vi "CPP-SolAEsaveTimeTraces.vi"() -> (5 "Plug in titles":string[](array[string]), 7 "Plug in values":string[](array[string]))   [LabVIEW 2021]
uses:
  Controls/File Header mode.ctl
  Globals/Meas_global.vi
panel:
  out "Data to save (ALL channels)":i32[](array[ring])
  # "Minimalist Save-All-Channels plugin, with options hard-coded to suit SolAE jobs\n\n\nYou Must have selected the \"Save Data\" option on the \nMeasurement Program for this vi to save time traces"
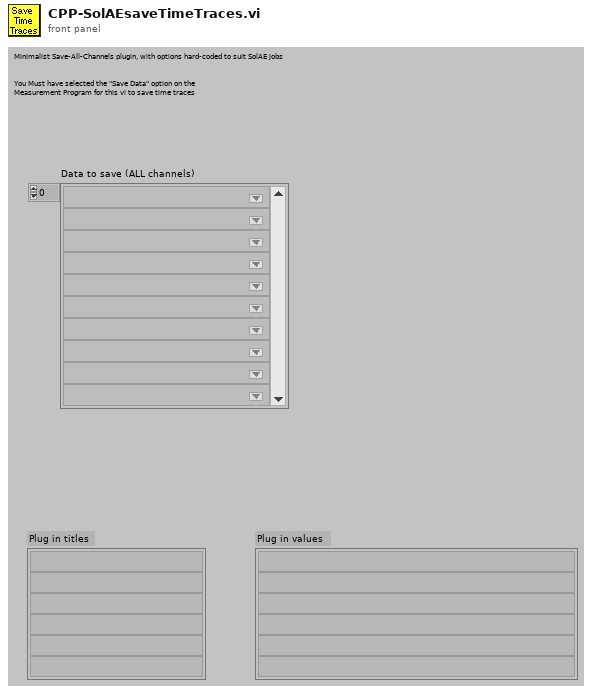
[diagram p1: front panel]
types:
  T1 = typedef "Analysis_info_cluster.ctl" = cluster{"Colour":u32, "Inst type":T2, "Inst name":string, "Symbol":string, "Code name":string, "Extra Info":string, "Inst Array":T3, "Extra Titles":string[], "Extra Values":string[], "U":dbl, "u^2":dbl, "u^3":dbl, "u^4":dbl, "Skew_u":dbl, "Kurt_u":dbl, "Sd Error in Mean":dbl, "% u'/U":dbl, "X":dbl, "Y":dbl, "Z":dbl, "Timescale integral Estimate":dbl, "Sd Error in Variance":dbl, "Calib File":path, "Calib Constants":dbl[], "Output Position":bool, "Stats":enum16{"None", "Basic", "Full"}, "Av Sampling Rate":dbl, "Av No of Samples":dbl, "Total Meas Time (s)":dbl, "ADAM Ch Name":string, "Max value":dbl, "Min value":dbl, "Req Sample Rate Hz":dbl, "Sync Delay Time (s)":dbl, "Ch No":i16, "Device":string, "Use Latest Calib":bool, "Port":string, "Metadata Ch Names":string[], "Metadata Ch Values":string[], "Label":string}
  T2 = typedef "Inst_type.ctl" = enum16{"Raw voltage", "Raw with zero offsetting", "Propeller anemometer", "Pressure Transducer", "Pitot-static tube", "Hot wire", "Cross wire 1", "Cross wire 2", "Generic Linear", "Generic Polynomial", "Generic BackPoly", "Fast FID", "Thermocouple", "Cold wire", "Pulsed Wire", "LDA Vel", "LDA Tran time", "LDA Arr time", "Microphone"}
  T3 = typedef "Instrument_Array.ctl" = enum16{"PWA", "LDA", "Analogue"}
  T4 = enum16{"Save no data", "Save data in new files", "Save data in existing files"}
  T5 = typedef "File Header mode.ctl" = enum16{"No Headers", "Headers in All files", "Separate Header File"}
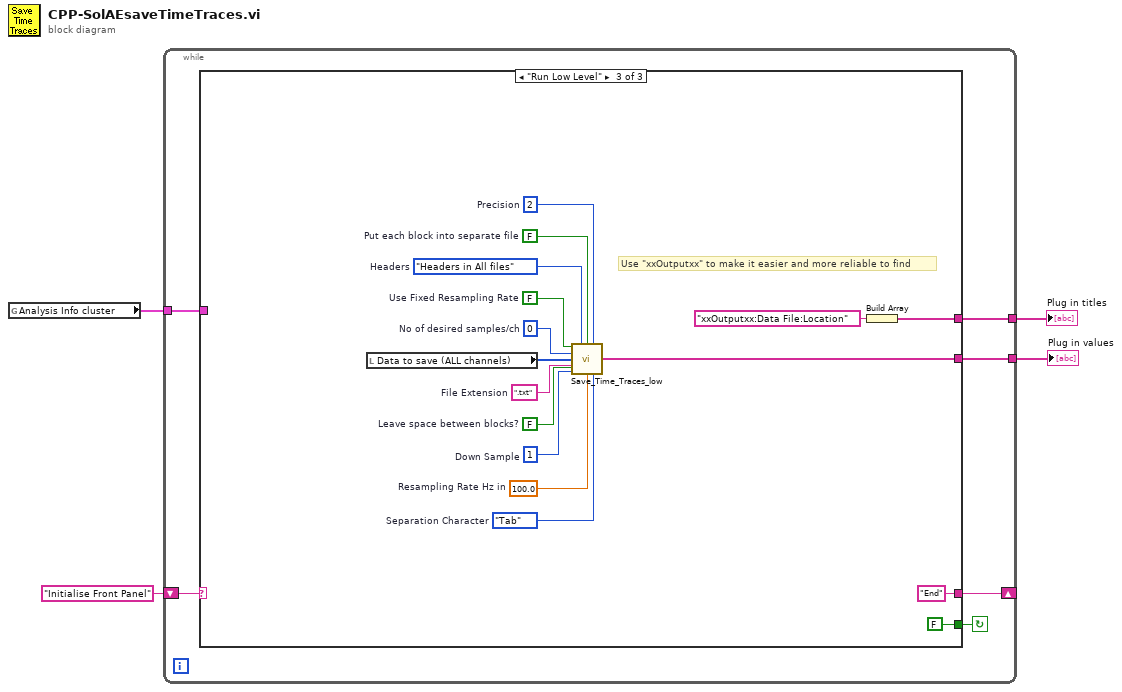
[diagram p0: block diagram]
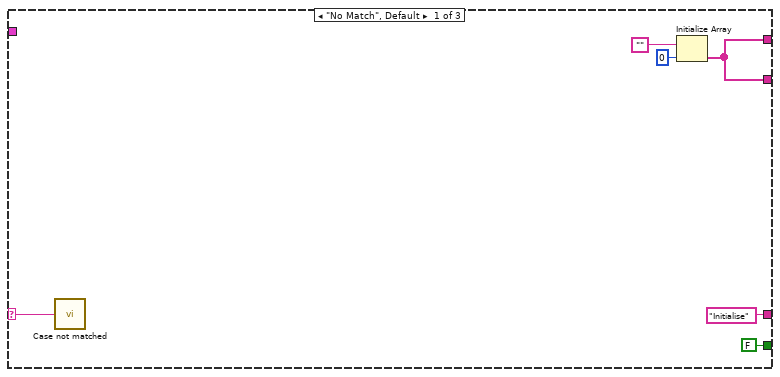
[diagram p2: hidden frame]
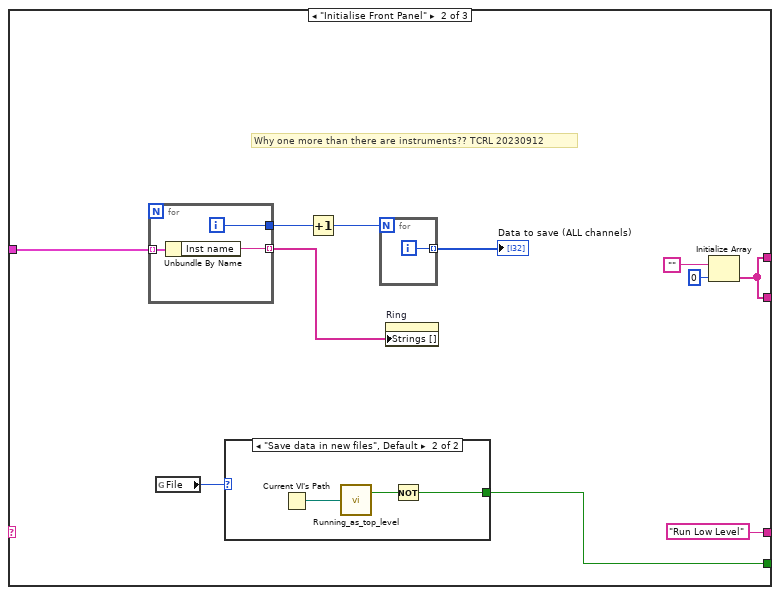
[diagram p3: hidden frame]
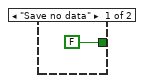
[diagram p4: hidden frame]
diagram:
  n1 = global read "Meas_global.vi" "Analysis Info cluster"() -> (w3:T1[])
  n2 = while {
    shift-left: "Initialise Front Panel" -> [w8]
    shift-right: [w9] -> _
    tunnel: w3 -> [w7]
    tunnel: [w6] -> w2
    tunnel: [w5] -> w1
    stop <- w10 continue-if-true
    n3 = case shown="\"Run Low Level\"" w8 {
      selector: w8 -> [w11 _ _]
      tunnel: [FALSE w23 FALSE] -> w10
      tunnel: ["Initialise" "Run Low Level" ("t") "End" ("t")] -> w9
      tunnel: w7 -> [_ w27 _]
      tunnel: [w12 w19 w38] -> w6
      tunnel: [w12 w19 w36] -> w5
      frame "No Match", Default {
        n4 = call "Case not matched.vi"("Case Name not Matched"=w11) -> ()
        n5 = Initialize Array("", 0) -> (w12:string[])
      }
      frame "Initialise Front Panel" {
        # "Why one more than there are instruments?? TCRL 20230912"
        n6 = for {
          tunnel: w27 -> [w35] mode=indexing
          tunnel: [w34] -> w26 mode=indexing
          tunnel: [w33] -> w22
          i -> [w33]
          n7 = Unbundle By Name(w35) -> ("Inst name"=w34:string)
        }
        n8 = global read "Meas_global.vi" "File"() -> (w24:T4)
        n9 = case shown="\"Save data in new files\", Default" w24 {
          tunnel: [FALSE w30] -> w23
          frame "Save no data" {
          }
          frame "Save data in new files", Default {
            n10 = Current VI's Path() -> (path=w31:path)
            n11 = call "Running_as_top_level.vi"("Vi path name"=w31) -> ("Top Level"=w32:bool)  [unwired: 1 out]
            n12 = Not(x=w32) -> (.not. x?=w30:bool)
          }
        }
        n13 = Increment(x=w22) -> (x+1=w18:i32)
        n14 = for {
          N: w18 -> [_]
          tunnel: [w28] -> w17 mode=indexing
          i -> [w28]
        }
        "Data to save (ALL channels)" <- w17
        n15 = property on="Ring" class="Ring (strict)"("Strings []"=w26) -> ()  [unwired: 2 in, 2 out]
        n16 = Initialize Array("", 0) -> (w19:string[])
      }
      frame "Run Low Level" {
        w39 = enum16{"Tab", "Comma"}."Tab"  # Separation Character
        w40 = 100.0  # Resampling Rate Hz in
        w41 = FALSE  # Leave space between blocks?
        w42 = 1  # Down Sample
        w43 = ".txt"  # File Extension
        w44 = 0  # No of desired samples/ch
        w45 = i16 2  # Precision
        w46 = FALSE  # Put each block into separate file
        w47 = File_Header_mode."Headers in All files"  # Headers
        w48 = FALSE  # Use Fixed Resampling Rate
        # "Use \"xxOutputxx\" to make it easier and more reliable to find"
        n17 = local read "Data to save (ALL channels)"() -> (w49:i32[])
        n18 = call "Save_Time_Traces_low.vi"("Use Fixed Resampling Rate"=w48, "Headers"=w47, "Put each block into separate file"=w46, "Precision"=w45, "No of desired samples/ch"=w44, "Data to save"=w49, "File Extension"=w43, "Down Sample"=w42, "Leave space between blocks?"=w41, "Resampling Rate Hz in"=w40, "Separation Character"=w39) -> ("Plug in values"=w38:string[])  [unwired: 3 in, 1 out]
        n19 = Build Array("xxOutputxx:Data File:Location") -> (w36:string[])
      }
    }
  }
  "Plug in values" <- w2
  "Plug in titles" <- w1
